vi "Anti-Spam Tester.vi"() -> ()   [LabVIEW 2023, in "Error Manager.lvlib" / "Anti-Spam Tester (AST).lvlib"]
uses:
  Anti-Spam Tester (AST).lvlib
  Error Manager.lvlib
  MHL Queue/AST MHL Queue.lvclass
  MHL Queue/Command (enum).ctl
  GUI refs - Input (cluster).ctl
  GUI refs - Buttons (cluster).ctl
  GUI refs (cluster).ctl
  Public API VIs/_TBD Pop-up New Error Dialogue Setting (enum).ctl
  <vilib>/Utility/sysdir.llb/System Directory Type.ctl
  Spam Mode (enum).ctl
  Spam Frequency (enum).ctl
  Spam Error Message Type (enum).ctl
panel:
  out "Error Logs Folder":path
  out "MHL iteration":i32
  in  "Error Message Type":T1=enum."Long Error Message"
  in  "How many error codes?":u32=1 caption="How many different error codes (different types of error)?" min=1 max=9
  in  "Spam Frequency":T2=enum."Every 100 ms"
  in  "Stop Spamming":bool
  in  "Start Spamming":bool
  in  "n (ms)":u32=5000 min=100 max=60000 step=100
  in  "Spam Mode":T3
  out "Error Out":errorcluster
  in  "Include call chain?":bool=TRUE
  in  "Show Error Manager GUI":bool
  in  "Exit Tester":bool
  out "EHL iteration":i32
  # "Anti-Spam Tester\nThis VI tests the Error Handler anti-spam functionality."
  # "Input"
  # "Control"
  # "Output"
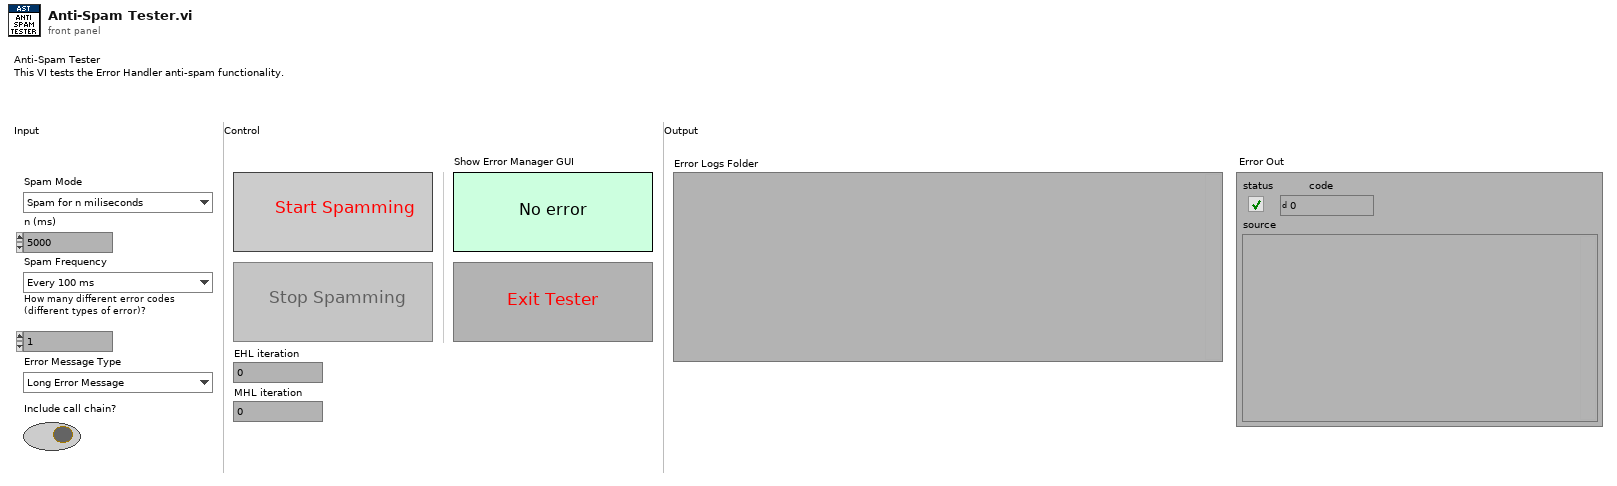
[diagram p1: front panel]
types:
  T1 = typedef "Error Manager.lvlib/Anti-Spam Tester (AST).lvlib/Spam Error Message Type (enum).ctl" = enum16{"Short Error Message", "Long Error Message"}
  T2 = typedef "Error Manager.lvlib/Anti-Spam Tester (AST).lvlib/Spam Frequency (enum).ctl" = enum16{"As fast as possible", "Every 1 ms", "Every 2 ms", "Every 5 ms", "Every 10 ms", "Every 20 ms", "Every 50 ms", "Every 100 ms", "Every 200 ms", "Every 500 ms", "Every 1000 ms"}
  T3 = typedef "Error Manager.lvlib/Anti-Spam Tester (AST).lvlib/Spam Mode (enum).ctl" = enum16{"Spam for n miliseconds", "Spam continuously"}
  T4 = typedef "System Directory Type.ctl" = i32
  T5 = typedef "Error Manager.lvlib/_TBD Pop-up New Error Dialogue Setting (enum).ctl" = enum16{"Pop-up New Error Dialogue", "Don't pop-up New Error Dialogue"}
  T6 = typedef "Error Manager.lvlib/Anti-Spam Tester (AST).lvlib/AST MHL Queue.lvclass/Command (enum).ctl" = enum16{"Init AST", "Close AST", "Config GUI - Init", "Config GUI - Spamming Has Started", "Config GUI - Spamming Has Stopped", "Spam"}
  T7 = typedef "Error Manager.lvlib/Anti-Spam Tester (AST).lvlib/GUI refs - Buttons (cluster).ctl" = cluster{"Start Spamming":refnum<vi>, "Stop Spamming":refnum<vi>}
  T8 = typedef "Error Manager.lvlib/Anti-Spam Tester (AST).lvlib/GUI refs - Input (cluster).ctl" = cluster{"Spam Mode":refnum<vi>, "n (ms)":refnum<vi>, "Spam Frequency":refnum<vi>, "How many error codes?":refnum<vi>, "Spam Error Message Type":refnum<vi>, "Include call chain?":refnum<vi>}
  T9 = typedef "Error Manager.lvlib/Anti-Spam Tester (AST).lvlib/GUI refs (cluster).ctl" = cluster{"Input":T8, "Buttons":T7}
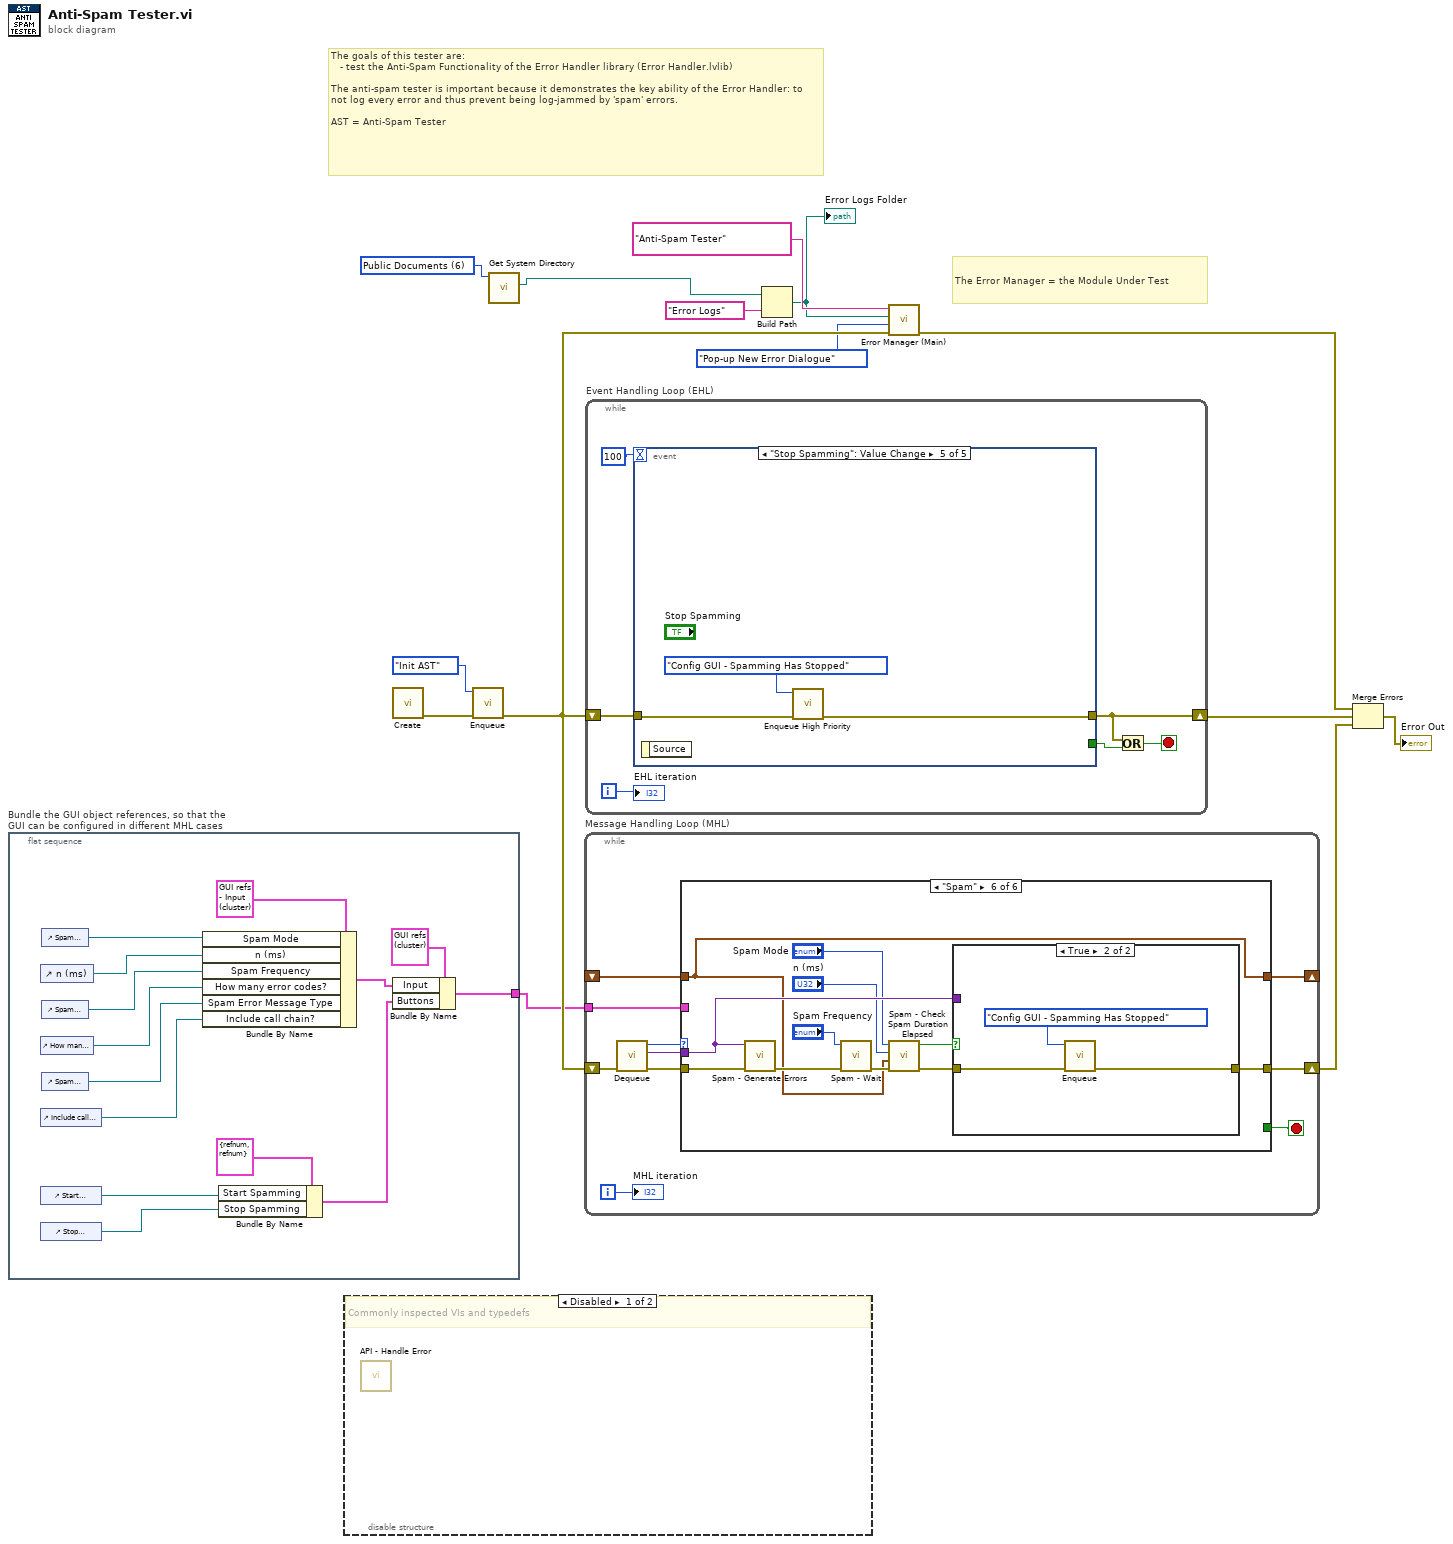
[diagram p0: block diagram]
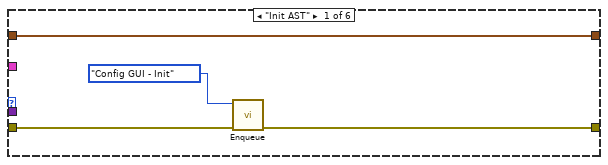
[diagram p3: hidden frame]
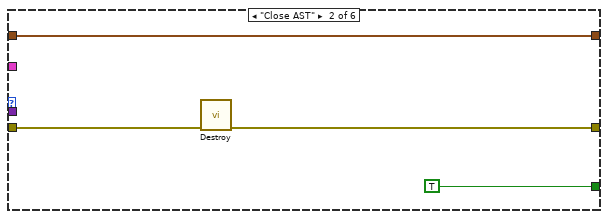
[diagram p4: hidden frame]
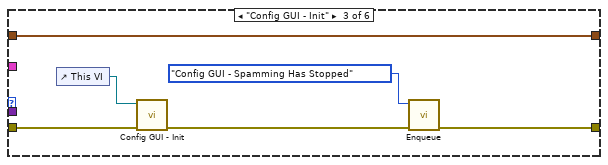
[diagram p5: hidden frame]
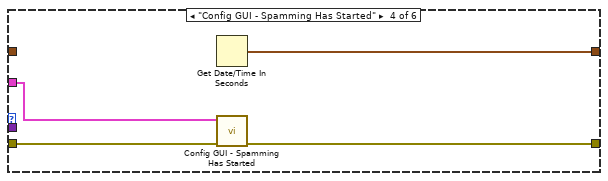
[diagram p6: hidden frame]
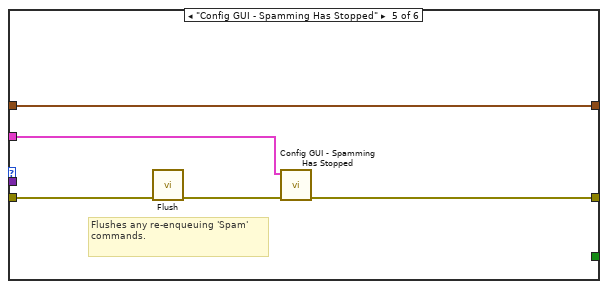
[diagram p7: hidden frame]
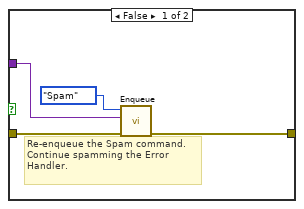
[diagram p8: hidden frame]
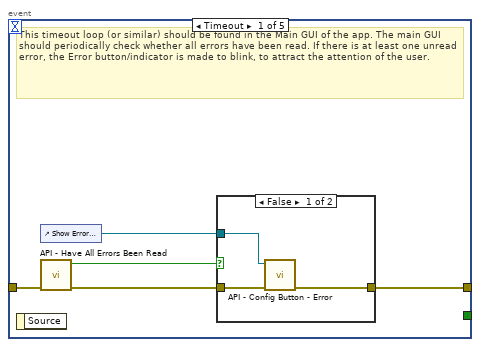
[diagram p9: hidden frame]
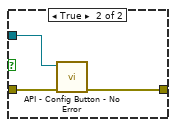
[diagram p10: hidden frame]
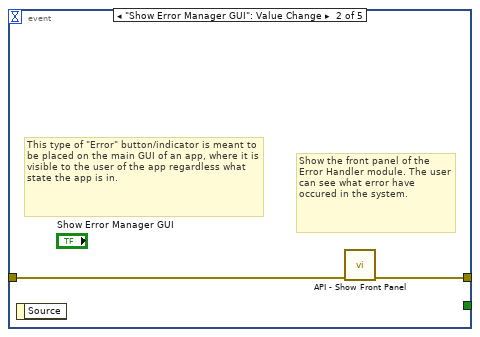
[diagram p11: hidden frame]
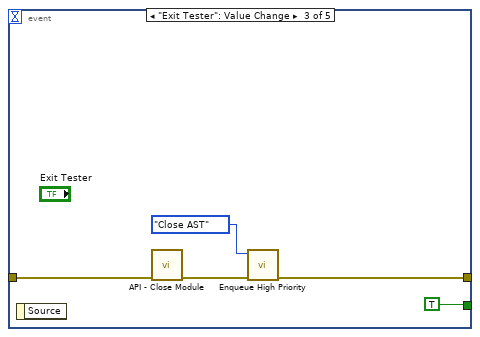
[diagram p12: hidden frame]
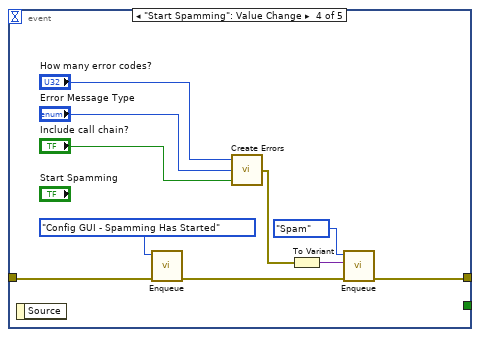
[diagram p13: hidden frame]
diagram:
  w1 = T4 6 items=["User Home"=0, "User Desktop"=1, "User Documents"=2, "User Application Data"=3, "User Preferences"=4, "User Temporary"=5, "Public Documents"=6, "Public Application Data"=7, "Public Preferences"=8, "Public Cache"=13, "System Core Libraries"=9, "System Installed Libraries"=10, "Application Files"=11, "Boot Volume Root"=12] ("system directory type")
  # "The Error Manager = the Module Under Test"
  # "The goals of this tester are:\n   - test the Anti-Spam Functionality of the Error Handler library (Error Handler.lvlib)\n\nThe anti-spam tester is important because it demonstrates the key ability of the Error Handler: to not log every error and thus prevent being log-jammed by 'spam' errors.\n\nAST = Anti-Spam Tester"
  n1 = flat-sequence "Bundle the GUI object references, so that the GUI can be configured in different MHL cases" {
    tunnel: [w15] -> w3
    frame #0 {
      n2 = control-ref of="n (ms)"() -> (w20:refnum<vi>)
      n3 = control-ref of="How many error codes?"() -> (w18:refnum<vi>)
      n4 = control-ref of="Include call chain?"() -> (w16:refnum<vi>)
      n5 = control-ref of="Start Spamming"() -> (w23:refnum<vi>)
      n6 = control-ref of="Stop Spamming"() -> (w22:refnum<vi>)
      n7 = control-ref of="Spam Mode"() -> (w21:refnum<vi>)
      n8 = control-ref of="Spam Frequency"() -> (w19:refnum<vi>)
      n9 = control-ref of="Spam Error Message Type"() -> (w17:refnum<vi>)
      n10 = Bundle By Name(cluster=T8 {"Spam Mode"=refnum, "n (ms)"=refnum, "Spam Frequency"=refnum, "How many error codes?"=refnum, "Spam Error Message Type"=refnum, "Include call chain?"=refnum} ("GUI refs - Input"), "Spam Mode"=w21, "n (ms)"=w20, "Spam Frequency"=w19, "How many error codes?"=w18, "Spam Error Message Type"=w17, "Include call chain?"=w16) -> (w26:T8)
      n11 = Bundle By Name(cluster=T7 {"Start Spamming"=refnum, "Stop Spamming"=refnum} ("GUI refs - Buttons"), "Start Spamming"=w23, "Stop Spamming"=w22) -> (w24:T7)
      n12 = Bundle By Name(cluster=T9 {"Input"={"Spam Mode"=refnum, "n (ms)"=refnum, "Spam Frequency"=refnum, "How many error codes?"=refnum, "Spam Error Message Type"=refnum, "Include call chain?"=refnum}, "Buttons"={"Start Spamming"=refnum, "Stop Spamming"=refnum}} ("GUI refs"), "Input"=w26, "Buttons"=w24) -> (w15:T9)
    }
  }
  n13 = disable-structure shown="Disabled" {
    frame Disabled {
      # "Commonly inspected VIs and typedefs"
      n14 = call "API - Handle Error.vi"() -> ()  [unwired: 11 in, 1 out]
    }
    frame Enabled {
    }
  }
  n15 = call "Create.vi"() -> ("error out"=w7:errorcluster)  [unwired: 11 in]
  n16 = call "Enqueue.vi"("error in (no error)"=w7, "Command"=Command_(enum)."Init AST") -> ("error out"=w5:errorcluster)  [unwired: 9 in]
  n17 = call <vilib>:"Get System Directory.vi"("system directory type"=w1) -> ("system directory"=w10:path)  [unwired: 10 in]
  n18 = while "Message Handling Loop (MHL)" {
    shift-right: [w35] -> w4
    shift-left: w5 -> [w38]
    tunnel: w3 -> [w32]
    shift-right: [w30] -> _
    shift-left: _ -> [w29]
    i -> [w33]
    stop <- w34 stop-if-true
    n19 = call "Dequeue.vi"("error in (no error)"=w38) -> ("error out"=w37:errorcluster, "Data"=w31:variant, "Command"=w36:T6)  [unwired: 8 in]
    n20 = case shown="\"Spam\"" w36 {
      tunnel: w37 -> [w41 w46 w49 w56 w61 w72]
      tunnel: [w40 w45 w50 w55 w60 w67] -> w35
      tunnel: [_ TRUE _ _ _ _] -> w34
      tunnel: w32 -> [_ _ _ w54 w59 _]
      tunnel: w31 -> [_ _ _ _ _ w66]
      tunnel: [w39 w43 w47 w53 w57 w63] -> w30
      tunnel: w29 -> [w39 w43 w47 _ w57 w63]
      frame "Init AST" {
        n21 = call "Enqueue.vi"("error in (no error)"=w41, "Command"=Command_(enum)."Config GUI - Init") -> ("error out"=w40:errorcluster)  [unwired: 9 in]
      }
      frame "Close AST" {
        n22 = call "Destroy.vi"("error in (no error)"=w46) -> ("error out"=w45:errorcluster)  [unwired: 8 in, 2 out]
      }
      frame "Config GUI - Init" {
        n23 = control-ref of="This VI"() -> (w48:refnum<vi>)
        n24 = call "Config GUI - Init.vi"("error in (no error)"=w49, "VI Reference"=w48) -> ("error out"=w51:errorcluster)  [unwired: 9 in]
        n25 = call "Enqueue.vi"("error in (no error)"=w51, "Command"=Command_(enum)."Config GUI - Spamming Has Stopped") -> ("error out"=w50:errorcluster)  [unwired: 9 in]
      }
      frame "Config GUI - Spamming Has Started" {
        n26 = Get Date/Time In Seconds() -> (seconds since 1Jan1904=w53:timestamp)
        n27 = call "Config GUI - Spamming Has Started.vi"("error in (no error)"=w56, "GUI refs"=w54) -> ("error out"=w55:errorcluster)  [unwired: 9 in]
      }
      frame "Config GUI - Spamming Has Stopped" {
        # "Flushes any re-enqueuing 'Spam' commands."
        n28 = call "Flush.vi"("error in (no error)"=w61) -> ("error out"=w58:errorcluster)  [unwired: 8 in, 2 out]
        n29 = call "Config GUI - Spamming Has Stopped.vi"("error in (no error)"=w58, "GUI refs"=w59) -> ("error out"=w60:errorcluster)  [unwired: 9 in]
      }
      frame "Spam" {
        n30 = call "Spam - Generate Errors.vi"("error in (no error)"=w72, "Variant"=w66) -> ("error out"=w69:errorcluster)  [unwired: 9 in]
        n31 = call "Spam - Wait.vi"("error in (no error)"=w69, "Spam Frequency"="Spam Frequency") -> ("error out"=w70:errorcluster)  [unwired: 9 in]
        n32 = call "Spam - Check Spam Duration Elapsed.vi"("error in (no error)"=w70, "Spam Started Timestamp"=w63, "n (ms)"="n (ms)", "Spam Mode"="Spam Mode") -> ("error out"=w68:errorcluster, "T = Spam duration has elapsed. Need to stop spamming."=w62:bool)  [unwired: 6 in]
        n33 = case shown="True" w62 {
          tunnel: w68 -> [w75 w78]
          tunnel: [w74 w77] -> w67
          tunnel: w66 -> [w73 _]
          frame False {
            # "Re-enqueue the Spam command. Continue spamming the Error Handler."
            n34 = call "Enqueue.vi"("error in (no error)"=w75, "Data"=w73, "Command"=Command_(enum)."Spam") -> ("error out"=w74:errorcluster)  [unwired: 8 in]
          }
          frame True {
            n35 = call "Enqueue.vi"("error in (no error)"=w78, "Command"=Command_(enum)."Config GUI - Spamming Has Stopped") -> ("error out"=w77:errorcluster)  [unwired: 9 in]
          }
        }
      }
    }
    "MHL iteration" <- w33
  }
  n36 = while "Event Handling Loop (EHL)" {
    shift-right: [w82] -> w13
    shift-left: w5 -> [w83]
    i -> [w85]
    stop <- w80 stop-if-true
    n37 = event shown="[4] \"Stop Spamming\": Value Change" {
      selector: _ -> [_ _ _ _ _]
      dyn-events: _ -> [_ _ _ _ _]
      timeout: 100 -> [_ _ _ _ _]
      tunnel: w83 -> [w90 w98 w102 w112 w115]
      tunnel: [w88 w97 w100 w109 w114] -> w82
      tunnel: [_ _ TRUE _ _] -> w81
      event Timeout {
        # "This timeout loop (or similar) should be found in the Main GUI of the app. The main GUI should periodically check whether all errors have been read. If there is at least one unread error, the Error button/indicator is made to blink, to attract the attention of the user."
        n38 = event-data() -> ()  [unwired: 1 in, 1 out]
        n39 = control-ref of="Show Error Manager GUI"() -> (w86:refnum<vi>)
        n40 = call "API - Have All Errors Been Read.vi"("error in"=w90) -> ("error out"=w89:errorcluster, "Have All Errors Been Read?"=w87:bool)  [unwired: 9 in]
        n41 = case shown="False" w87 {
          tunnel: [w91 w95] -> w88
          tunnel: w89 -> [w92 w96]
          tunnel: w86 -> [w93 w94]
          frame False {
            n42 = call "API - Config Button - Error.vi"("error in"=w92, "Error Button"=w93) -> ("error out"=w91:errorcluster)  [unwired: 9 in]
          }
          frame True {
            n43 = call "API - Config Button - No Error.vi"("error in"=w96, "Error Button"=w94) -> ("error out"=w95:errorcluster)  [unwired: 9 in]
          }
        }
      }
      event "Show Error Manager GUI": Value Change {
        # "This type of \"Error\" button/indicator is meant to be placed on the main GUI of an app, where it is visible to the user of the app regardless what state the app is in."
        # "Show the front panel of the Error Handler module. The user can see what error have occured in the system."
        n44 = event-data() -> ()  [unwired: 1 in, 1 out]
        n45 = call "API - Show Front Panel.vi"("error in"=w98) -> ("error out"=w97:errorcluster)  [unwired: 10 in]
      }
      event "Exit Tester": Value Change {
        n46 = event-data() -> ()  [unwired: 1 in, 1 out]
        n47 = call "API - Close Module.vi"("error in"=w102) -> ("error out"=w103:errorcluster)  [unwired: 10 in]
        n48 = call "Enqueue High Priority.vi"("error in (no error)"=w103, "Command"=Command_(enum)."Close AST") -> ("error out"=w100:errorcluster)  [unwired: 9 in]
      }
      event "Start Spamming": Value Change {
        n49 = event-data() -> ()  [unwired: 1 in, 1 out]
        n50 = call "Enqueue.vi"("error in (no error)"=w112, "Command"=Command_(enum)."Config GUI - Spamming Has Started") -> ("error out"=w110:errorcluster)  [unwired: 9 in]
        n51 = call "Create Errors.vi"("Include call chain?"="Include call chain?", "Error Message Type"="Error Message Type", "Number of different error codes"="How many error codes?") -> ("Errors"=w108:errorcluster[])
        n52 = To Variant(anything=w108) -> (Variant=w107:variant)
        n53 = call "Enqueue.vi"("error in (no error)"=w110, "Data"=w107, "Command"=Command_(enum)."Spam") -> ("error out"=w109:errorcluster)  [unwired: 8 in]
      }
      event "Stop Spamming": Value Change {
        n54 = event-data() -> ()  [unwired: 1 in, 1 out]
        n55 = call "Enqueue High Priority.vi"("error in (no error)"=w115, "Command"=Command_(enum)."Config GUI - Spamming Has Stopped") -> ("error out"=w114:errorcluster)  [unwired: 9 in]
      }
    }
    n56 = Or(x=w82, y=w81) -> (x .or. y?=w80:bool)
    "EHL iteration" <- w85
  }
  n57 = Build Path(base path=w10, name or relative path="Error Logs") -> (appended path=w8:path)
  "Error Logs Folder" <- w8
  n58 = call "Error Manager (Main).vi"("Error In"=w5, 9:_TBD_Pop-up_New_Error_Dialogue_Setting_(enum)."Pop-up New Error Dialogue" ("Pop-up New Error Dialogue Setting (Default = Pop-up Dialogue)"), 10:w8, "Settings Filepath"="Anti-Spam Tester" ("Jig Name or Acronym")) -> ("Error Out"=w14:errorcluster)  [unwired: 7 in]
  n59 = Merge Errors(w14, w13, w4) -> (→"Error Out":errorcluster)
